vi "Lake Shore 336 Write Curve.vi"(0 "VISA resource name":refnum<visa-resource-name>) -> ()   [LabVIEW 2019]
doc: "This example VI demonstrates the proper use of the Configure Curve Header and Configure Curve Point VIs. It allows the user to write a curve header, a curve point, of both."
uses:
  Lake Shore 336.lvlib
panel:
  in  "Temperature Value (0.0000)":dbl format="%.4f"
  in  "Index (1)":dbl=1.0
  in  "Units Value (0.00000)":dbl format="%.5f"
  in  "Coefficient (1:Negative)":u16(ring)=1 items=["Negative"=1, "Positive"=2]
  in  "Curve Serial Number (\"\")":string
  in  "Curve (21)":dbl=21.0
  in  "Curve Name (\"\")":string
  in  "Limit Value (375.000)":dbl=375.0 format="%.3f"
  in  "Curve Data Format (1:mV/K)":u16(ring)=1 items=["mV/K"=1, "V/K"=2, "Ohms/K"=3, "Log Ohms/K"=4]
  in  "Configure Curve Point\n (1: Don't Configure)":u16(ring) items=["Configure", "Don't Configure"]
  in  "Configure Curve Header (1: Don't Configure)":u16(ring) items=["Configure", "Don't Configure "]
  in  "Serial Configuration":T1={"Baud Rate"=57600, "Parity"=1, "Data Bits"=7, "Stop Bits"=10, "Flow Control"=0} {"Flow Control" items=["None", "XON/XOFF", "RTS/CTS", "XON/XOFF & RTS/CTS", "DTR/DSR", "XON/XOFF & DTR/DSR"]; "Stop Bits" items=["1.0"=10, "1.5"=15, "2.0"=20]; "Data Bits" items=["7"=7, "8"=8]; "Parity" items=["None", "Odd", "Even", "Mark", "Space"]; "Baud Rate" items=["300"=300, "600"=600, "1200"=1200, "2400"=2400, "4800"=4800, "9600"=9600, "19200"=19200, "38400"=38400, "57600"=57600]}
  # "(c) 2009 Lake Shore Cryotronics Inc.  ALL RIGHTS RESERVED."
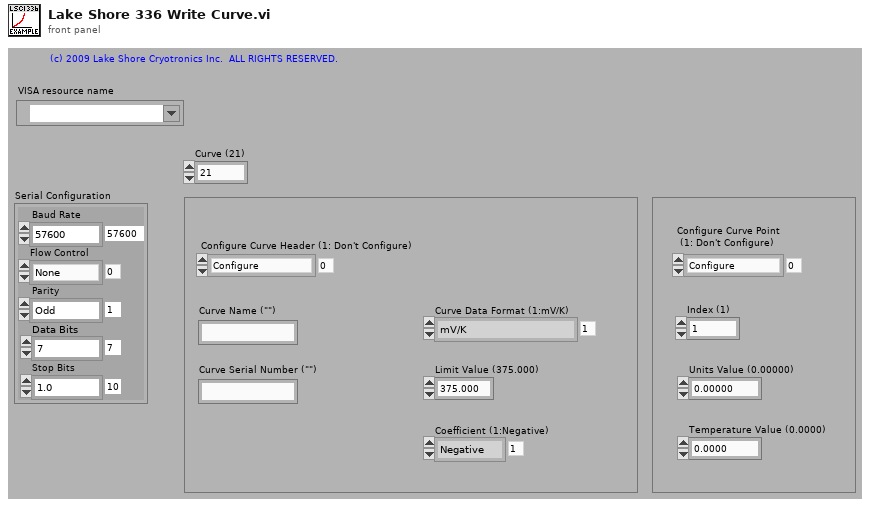
[diagram p1: front panel]
types:
  T1 = cluster{"Baud Rate":u32, "Parity":u16, "Data Bits":u16, "Stop Bits":u16, "Flow Control":u16}
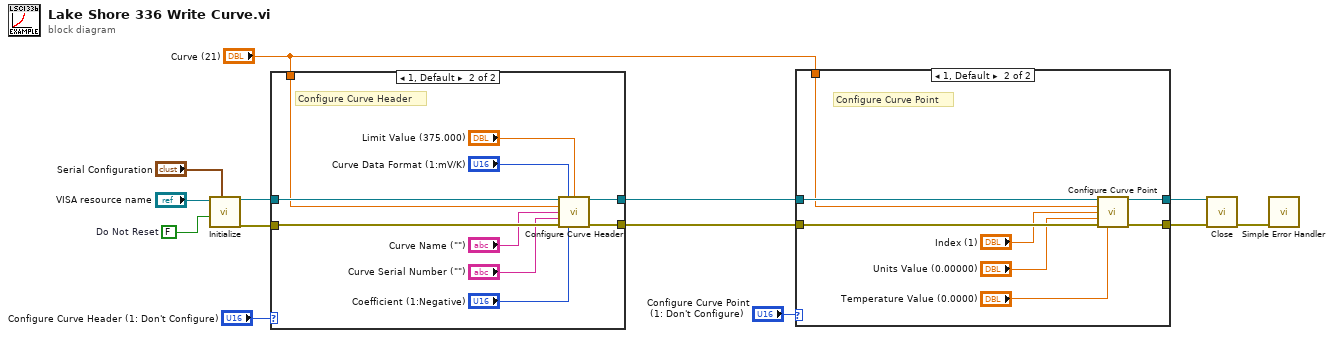
[diagram p0: block diagram]
diagram:
  w11 = FALSE  # Do Not Reset
  n1 = call "Initialize.vi"("Serial Configuration"="Serial Configuration", "Reset (True)"=w11, "VISA resource name"="VISA resource name") -> ("error out"=w6:errorcluster, "VISA resource name out"=w7:refnum<visa-resource-name>)  [unwired: 7 in]
  n2 = case shown="1, Default" "Configure Curve Header (1: Don't Configure)" {
    tunnel: w7 -> [w15 w25]
    tunnel: w6 -> [w14 w24]
    tunnel: [w15 w23] -> w5
    tunnel: [w14 w22] -> w4
    tunnel: "Curve (21)" -> [_ w21]
    frame 0 {
      # "Do Not Configure Curve Header"
    }
    frame 1, Default {
      # "Configure Curve Header"
      n3 = call "Configure Curve Header.vi"("VISA resource name"=w25, "Curve Data Format (1:mV/K)"="Curve Data Format (1:mV/K)", "Limit Value (375.000)"="Limit Value (375.000)", "Curve (21)"=w21, "Curve Name (\"\")"="Curve Name (\"\")", "Curve Serial Number (\"\")"="Curve Serial Number (\"\")", "error in (no error)"=w24, "Coefficient (1:Negative)"="Coefficient (1:Negative)") -> ("VISA resource name out"=w23:refnum<visa-resource-name>, "error out"=w22:errorcluster)  [unwired: 6 in]
    }
  }
  n4 = case shown="1, Default" "Configure Curve Point\n (1: Don't Configure)" {
    tunnel: w5 -> [w27 w34]
    tunnel: w4 -> [w26 w35]
    tunnel: [w27 w33] -> w3
    tunnel: [w26 w32] -> w2
    tunnel: "Curve (21)" -> [_ w31]
    frame 0 {
      # "Do Not Configure Curve Point"
    }
    frame 1, Default {
      # "Configure Curve Point"
      n5 = call "Configure Curve Point.vi"("VISA resource name"=w34, "Curve (21)"=w31, "Index (1)"="Index (1)", "Units Value (0.00000)"="Units Value (0.00000)", "error in (no error)"=w35, "Temperature Value (0.0000)"="Temperature Value (0.0000)") -> ("VISA resource name out"=w33:refnum<visa-resource-name>, "error out"=w32:errorcluster)  [unwired: 8 in]
    }
  }
  n6 = call "Close.vi"("error in (no error)"=w2, "VISA resource name"=w3) -> ("error out"=w12:errorcluster)  [unwired: 9 in]
  n7 = call <vilib>:"Simple Error Handler.vi"("error in (no error)"=w12) -> ()  [unwired: 4 in, 5 out]
